vi "PositionCtrl_DriveFwdBck_Example.vi"() -> ()   [LabVIEW 2019]
uses:
  <vilib>/Rock Robotics/WPI/ThirdParty/JAS_Junk/TrajLib/SlewRateLimiter_New.vi
  <vilib>/Rock Robotics/WPI/ThirdParty/JAS_Junk/TrajLib/SlewRateLimiter_Reset.vi
  <vilib>/Rock Robotics/WPI/ThirdParty/JAS_Junk/TrajLib/SlewRateLimiter_Calculate.vi
  <vilib>/Rock Robotics/WPI/ThirdParty/JAS_Junk/TrajLib/SlewRateLimiter_SetRate.vi
  <vilib>/Rock Robotics/WPI/ThirdParty/JAS_Junk/TrajLib/Util_GetTime.vi
  <vilib>/Rock Robotics/WPI/ThirdParty/JAS_Junk/TrajLib/VI/Util_GetTime_U32.vi
  <vilib>/Rock Robotics/WPI/ThirdParty/JAS_Junk/TrajLib/VI/Util_GetTime_U64.vi
  <vilib>/Rock Robotics/WPI/ThirdParty/JAS_Junk/TrajLib/Trajectory_Library.lvlib
panel:
  in  "Tab Control":enum32{"Operation", "Tuning"}(tab)
  out "Targets along the way":cluster{dbl, "PositionError":dbl, dbl}(graph)
  in  "SP - Desired Position\n (Inch)":dbl(slide) scale=-10.0..350.0
  out "PV - Current Position\n (Inch)":dbl(slide) scale=-10.0..350.0
  out "Goal":T1(graph)
  out "Motor Output":dbl format="%13.3f"
  out "AtSetpoint":bool
  out "AtGoal":bool
  out "PositionError  \n(Inch)":dbl format="%13.2f"
  out "Velocity  (Inch/Sec)":dbl format="%13.2f"
  out "Velocity  \n(Inch/Sec) 2":dbl format="%13.2f"
  in  "Position Threshold\n(inch)":dbl=50.0 format="%#_13g"
  in  "Ki":dbl=0.15 format="%#_13g"
  in  "Kd":dbl format="%#_13g"
  in  "Output Deadband\n(mot units)":dbl=0.08 format="%#_13g"
  in  "Max Accel  (Inch/Sec^2)":dbl=60.0 format="%#_13g"
  in  "Position\nDeadband (Inch)":dbl=0.08 format="%#_13g"
  # "Position has hard limit\n at -5 and 300 inches"
  # "SET THESE BEFORE EXECUTING THIS PROGRAM."
  # "PID Tuning Parameters"
  # "Desired Profile Performance"
  # "Desired On Target Tolerance"
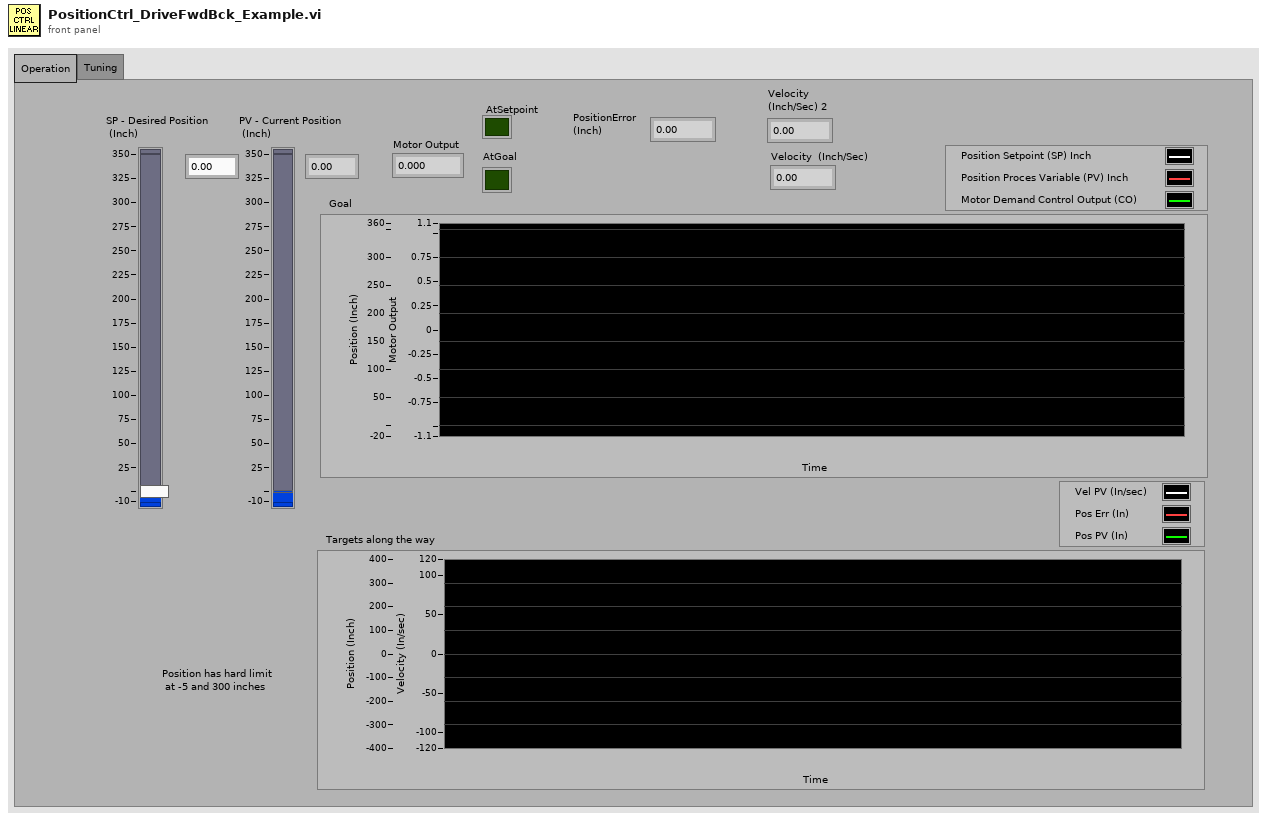
[diagram p1: front panel]
types:
  T1 = cluster{"SP - Desired Position\n (Inch)":dbl, "upper limit":dbl, "upper limit":dbl}
  T2 = typedef "Trajectory_Library.lvlib/PosCtrl_Tuning_Type.ctl" = cluster{"Slope":dbl, "Offset":dbl, "Error Deadband":dbl, "At Reference Count":i32, "Negate Output":bool, "Max Allowd Position":dbl, "Min Allowd Position":dbl}
  T3 = cluster{"SP - Desired Position\n (Inch)":dbl, dbl, "Result":dbl}
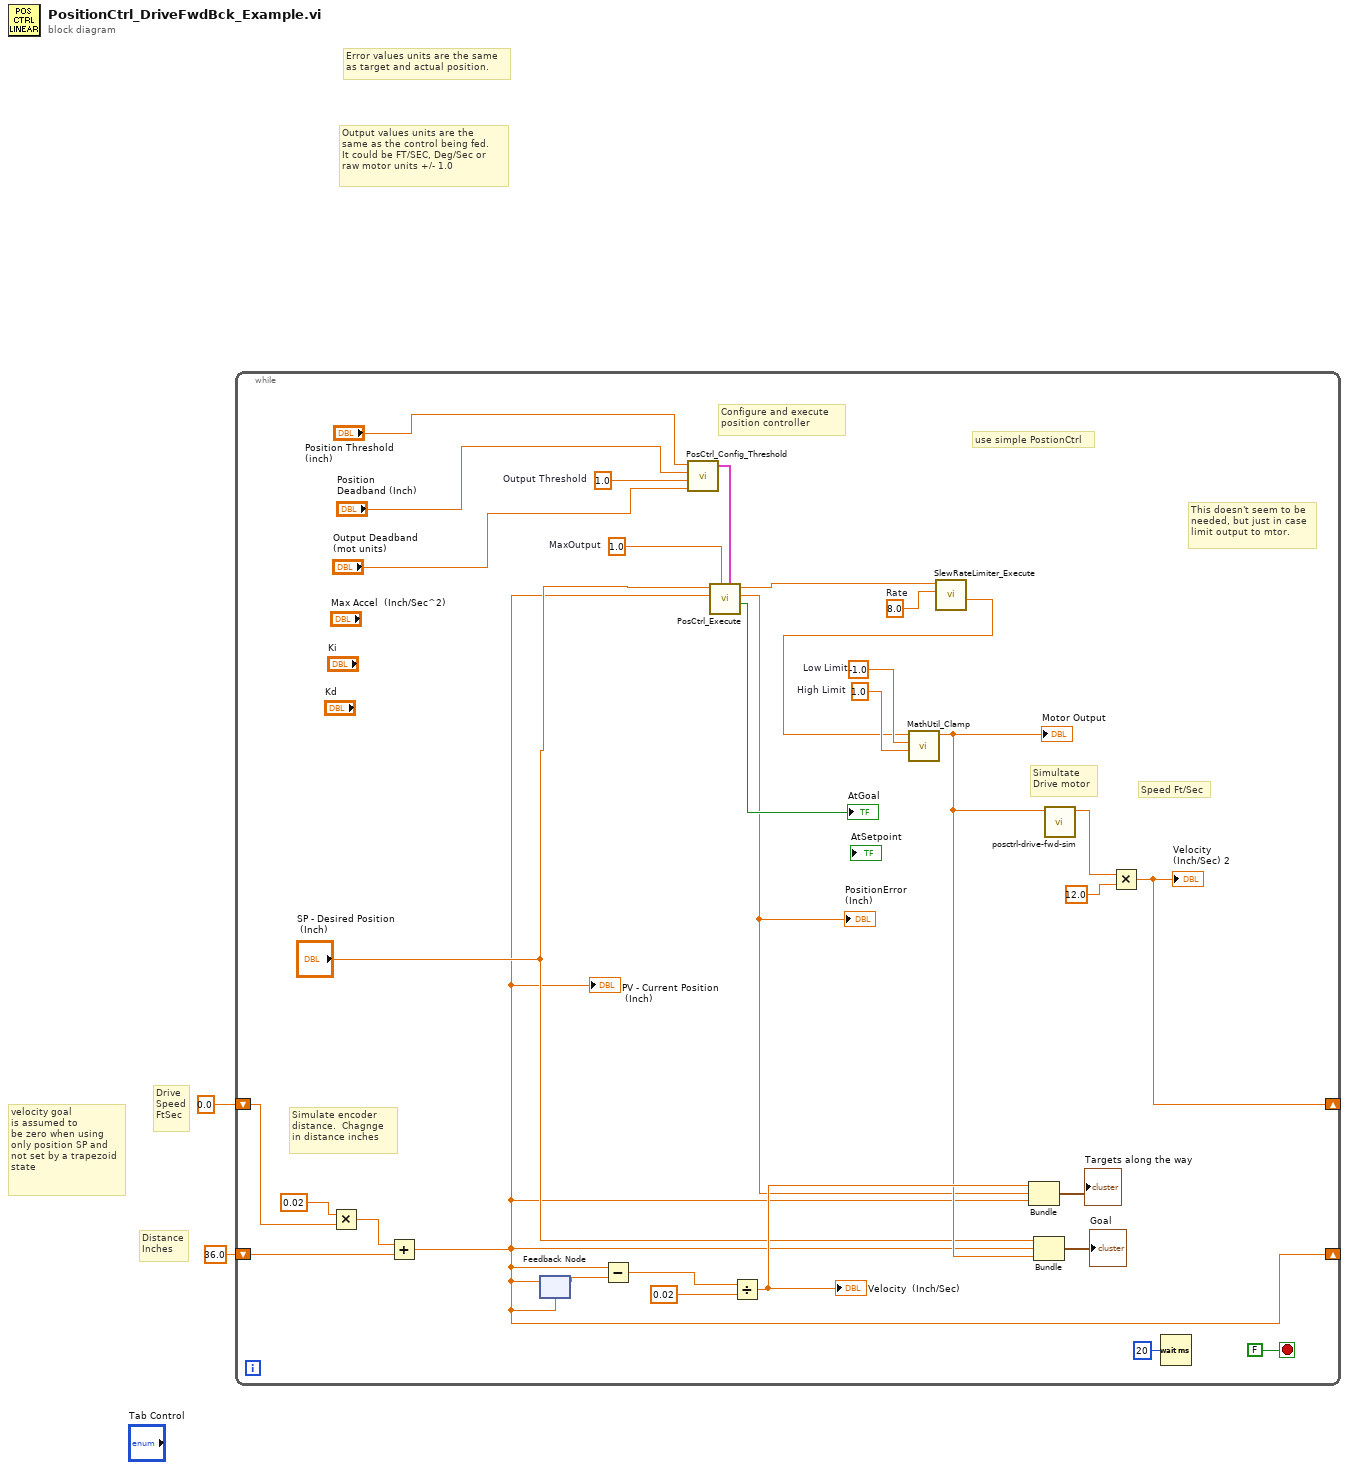
[diagram p0: block diagram]
diagram:
  # "Output values units are the\nsame as the control being fed.  \nIt could be FT/SEC, Deg/Sec or\nraw motor units +/- 1.0"
  # "Error values units are the same \nas target and actual position."
  # "velocity goal\nis assumed to \nbe zero when using\nonly position SP and\nnot set by a trapezoid\nstate"
  # "Distance\nInches"
  # "Drive\nSpeed\nFtSec"
  n1 = while {
    shift-right: [w11] -> _
    shift-left: 36.0 ("upper limit") -> [w25]
    shift-right: [w16] -> _
    shift-left: 0.0 ("upper limit") -> [w22]
    stop <- FALSE stop-if-true
    w6 = 8.0  # Rate
    w14 = 1.0  # MaxOutput
    w13 = 1.0  # Output Threshold
    w21 = 1.0  # High Limit
    w20 = -1.0  # Low Limit
    # "Configure and execute \nposition controller"
    # "This doesn't seem to be\nneeded, but just in case\nlimit output to mtor."
    # "use simple PostionCtrl"
    # "Speed Ft/Sec"
    # "Simultate \nDrive motor"
    # "Simulate encoder \ndistance.  Chagnge \nin distance inches"
    n2 = Multiply(x=0.02 ("value"), y=w22) -> (x*y=w27:dbl)
    n3 = Add(x=w27, y=w25) -> (x+y=w11:dbl)
    "PV - Current Position\n (Inch)" <- w11
    n4 = feedback-in #1(w11) -> ()
    n5 = feedback #1(w11) -> (w31:dbl)
    n6 = Subtract(x=w11, y=w31) -> (x-y=w30:dbl)
    n7 = call <vilib>:"PosCtrl_Config_Threshold.vi"("Output Deadband"="Output Deadband\n(mot units)", "Output Threshold"=w13, "ErrorDeadband"="Position\nDeadband (Inch)", "ErrorThreshold"="Position Threshold\n(inch)") -> ("PosCtrl_Config_Params"=w15:T2)  [unwired: 7 in]
    n8 = call <vilib>:"PosCtrl_Execute.vi"("PosCtrl_Config_Params"=w15, "MaxOutput"=w14, "CurrentPosition"=w11, "TargetPosition"="SP - Desired Position\n (Inch)") -> ("OnTarget"=→"AtGoal":bool, "PositionError"=w3:dbl, "Output"=w5:dbl)  [unwired: 5 in]
    "PositionError  \n(Inch)" <- w3
    n9 = Divide(x=w30, y=0.02) -> (x/y=w23:dbl)
    "Velocity  (Inch/Sec)" <- w23
    n10 = call <vilib>:"SlewRateLimiter_Execute.vi"("PositiveRate"=w6, "Input"=w5) -> ("Output"=w4:dbl)  [unwired: 8 in, 1 out]
    n11 = call <vilib>:"MathUtil_Clamp.vi"("High Limit"=w21, "Low Limit"=w20, "Value"=w4) -> ("Result"=w19:dbl)  [unwired: 8 in]
    "Motor Output" <- w19
    n12 = Bundle(w23, "PositionError"=w3, w11) -> (→"Targets along the way":cluster{dbl, "PositionError":dbl, dbl})  [unwired: 1 in]
    n13 = Bundle("SP - Desired Position\n (Inch)"="SP - Desired Position\n (Inch)", w11, "Result"=w19) -> (→"Goal":T3)  [unwired: 1 in]
    n14 = call "posctrl-drive-fwd-sim.vi"("Motor Demand"=w19) -> ("Drive Speed Ft/Sec"=w18:dbl)  [unwired: 10 in]
    n15 = Multiply(x=w18, y=12.0) -> (x*y=w16:dbl)
    "Velocity  \n(Inch/Sec) 2" <- w16
    n16 = Wait (ms)(milliseconds to wait=u32 20) -> ()  [unwired: 1 out]
  }
